vi "Write Warm-Up Time.vi"(8 "error in (no error)":errorcluster, 10 "Warm-Up Time":dbl, 11 "Abstract Display in":refnum<class "Abstract Display.lvclass">) -> (0 "error out":errorcluster, 3 "Abstract Display out":refnum<class "Abstract Display.lvclass">)   [LabVIEW 2013, in "Display Panel.lvlib" / "Abstract Display.lvclass"]
uses:
  Abstract Display.lvclass
  Abstract Display.lvclass/Abstract Display.ctl
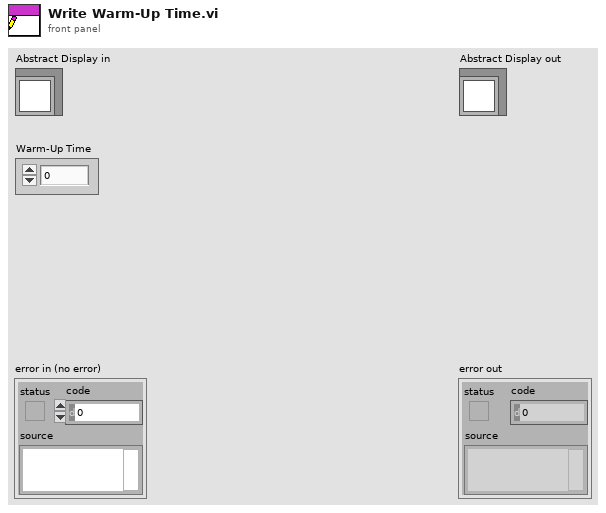
[diagram p1: front panel]
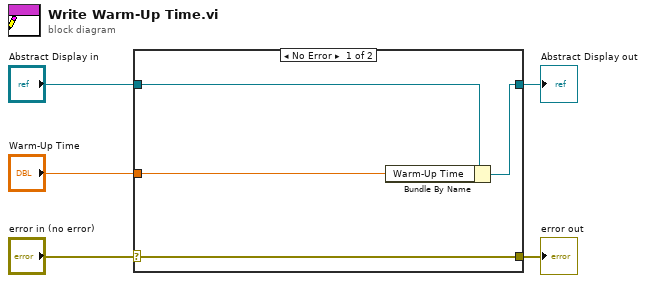
[diagram p0: block diagram]
diagram:
  n1 = case shown="No Error" "error in (no error)" {
    selector: "error in (no error)" -> [w9 w10]
    tunnel: [w9 w10] -> w4
    tunnel: [w7 w11] -> w2
    tunnel: "Abstract Display in" -> [w8 w11]
    tunnel: "Warm-Up Time" -> [w6 _]
    frame No Error {
      n2 = Bundle By Name(cluster=w8, "Warm-Up Time"=w6) -> (w7:refnum<class "Abstract Display.lvclass">)
    }
    frame Error {
    }
  }
  "error out" <- w4
  "Abstract Display out" <- w2
